vi "optionsAcq_spectrumSmoothing.vi"(0 "reference":refnum<class "OSA300.lvclass">, 2 "smoothing":T1, 4 "readWrite":enum16{"read", "write"}(ring), 5 "error in (no error)":errorcluster, 6 "width":u16, 7 "ignore range violation (false)":bool, 8 "nrOfPasses":u16) -> (10 "nrOfPasses out":u16, 12 "width out":u16, 14 "duplicate reference":refnum<class "OSA300.lvclass">, 15 "status":string, 16 "smoothing out":T1, 19 "error out":errorcluster)   [LabVIEW 2010, in "OSA300.lvclass"]
uses:
  OSA300.lvclass
  _misc/Thorlabs_FTS_misc.llb/interferogram_smoothing.ctl
  OSA.lvclass
  OSA300.lvclass/OSA300.ctl
  _OSAchannel_class/OSAchannel.lvclass
  _dll/LVLib/FTSLib.lvlib
  OSA20X_misc.lvlib
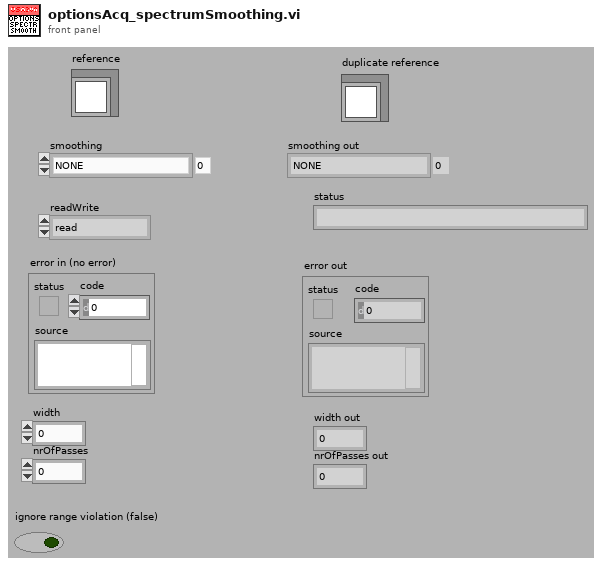
[diagram p1: front panel]
types:
  T1 = typedef "OSA20X_misc.lvlib/interferogram_smoothing.ctl" = enum16{"NONE", "BINOMIAL", "SAVITSKY_GOLAY", "FOURIER", "MOVING_AVERAGE", "GAUSSIAN"}
  T2 = typedef "OSA20X_misc.lvlib/channelType_spectrum.ctl" = enum16{"SINGLE CHANNEL", "STICHED"}
  T3 = typedef "OSA20X_misc.lvlib/amplifier_sort.ctl" = enum16{"amp_unknown", "amp_se_8", "amp_se_12_lg", "amp_se_12", "amp_se_16", "amp_diff_8", "amp_diff_12_lg", "amp_diff_12_ir", "amp_diff_16", "amp_other", "amp_other_2"}
  T4 = typedef "OSA20X_misc.lvlib/detector_sort.ctl" = enum16{"unknown", "Silicon", "Silicon PIN", "Silicon MPPC", "InGaAs", "InGaAs ext low", "InGaAs ext high", "InAs", "InAsSb", "InSb", "MCT", "other", "other2", "other3"}
  T5 = typedef "OSA20X_misc.lvlib/PDTemperatureMode.ctl" = enum16{"cool: better sensitivity/noise floor", "warm: extended wl range"}
  T6 = cluster{"waveMin (cm-1)":sgl, "waveMax (cm-1)":sgl, "gainOffset_auto":bool, "gain":i32, "gain levels nr":u16, "offset":i32, "offset max":u16, "damper available":bool, "damper active":bool, "amplifier sort":T3, "detector sort":T4, "channelIdx global":u16, "spectrIdx":u16, "waveMeter on":bool, "ref gainLevels rel.":refnum<data-value>, "intfgrm_smooth_width":u16, "intfgrm_smooth_nrOfPasses":u16, "intfgrm_smooth":T1, "adc #bits":u16, "temp Variable":bool, "spectr_smooth":T1, "spectr_smooth_width":u16, "spectr_smooth_nrOfPasses":u16, "PD sensitivity mode":T5}
  T7 = typedef "OSA.lvclass/ObjectAttributes.ctl" = cluster{"Stop":bool, "dataType":T8, "spectrometerIdx":u16, "buffer size interferogram":i32, "interferogram":cluster{"new":bool, "plot_x_ min":sgl, "plot_x_max":sgl, "plot_y_min":sgl, "plot_y_max":sgl, "Graph Intrfrgrm":T9, "timeStamp":u32, "signal (%)":dbl, "traces":cluster{"idx":u32, "broadBand":bool, "monoChromatic":bool, "peakToPeakSignal":dbl, "peakToPeakPos":dbl}[], "traces idx last":i32}, "spectrum":cluster{"new":bool, "plot_x_min":sgl, "plot_x_max":sgl, "plot_unit_x":T10, "plot_unit_y":T11, "plot_y_min":sgl, "plot_y_max":sgl, "Graph Spectrum":T9, "timeStamp":u32, "X_VAL_OPTIONS":enum16{"MIN_MAX", "ARRAY"}, "traces":cluster{"idx":u32}[], "traces idx last":i32}, "Thorlabs_OSA_64.lvclass:queue_action.ctlqueue ref":refnum<queue>, "action":T12, "plot zoom step":dbl, "buffer semaphore":T13, "acq stopped":bool, "dataType active":T8, "temperature (degr C)":sgl, "pressure (hPa)":sgl, "rel humidity (%)":sgl, "settings":cluster{"resolution":T14, "sensitivity":T15, "Average":bool, "average nr":u32, "apodisation":T16, "acq delay (ms)":u32, "airMesure":T17, "wmtr on":bool, "intfgrm_smooth_width":u16, "intfgrm_smooth_nrOfPasses":u16, "intfgrm_smooth":T1, "phaseCorrection":T18, "zeroFill":u8, "spectr_smooth":T1, "spectr_smooth_width":u16, "spectr_smooth_nrOfPasses":u16, "resolution (/cm)":sgl, "REF wavelength, (nm)":dbl, "gain_idx":u16, "gainAuto":bool, "gain_relative":dbl, "PD sensitivity mode":T5, "PD senseMode implemented":bool, "SensorTemperature implemented":bool, "SensorPressure implemented":bool, "SensorHumidity implemented":bool}, "peaks position":sgl[], "peaks width":sgl[], "peaks height":sgl[], "peaks max nr":u32, "peaks latest nr":i32, "peaks new":bool, "power":dbl, "power new":bool, "path":string, "wavelength (WNr)":dbl, "wavelength new":bool, "buffer size spectrum":i32, "status":string, "VI reference":refnum<vi>, "funcPointer":u64, "libraryPointer":u64, "singleAcquisition":bool, "coherenceLength (cm)":dbl, "coherenceLength new":bool, "spectrometer model":string, "spectrometer serial nr":string, "peaks thld left":sgl[], "peaks thld right":sgl[], "coherenceLength error (cm)":dbl, "ADC bits":u16, "peaks position centroid":sgl[], "peaks height centroid":sgl[], "OSA series":T19, "channel index spectrum":u16, "spectrometer rangeLow, (/cm)":dbl, "spectrometer rangeHigh, (/cm)":dbl, "channel index interferogram":u16}
  T8 = typedef "OSA.lvclass/acq_dataType.ctl" = enum16{"none", "interferogram", "spectrum"}
  T9 = typedef "OSA.lvclass/graph_intensity.ctl" = refnum<vi>
  T10 = typedef "OSA.lvclass/spectrum_x_unit.ctl" = enum16{"wavenr/cm", "THz", "eV", "nm_air", "nm_vac"}
  T11 = typedef "OSA.lvclass/y_unit.ctl" = enum16{"ADC counts", "dBm pwr absolute", "dBm pwr density", "mW pwr absolute", "mW pwr density"}
  T12 = typedef "OSA.lvclass/queue_action.ctl" = enum16{"none", "stop", "GUI_plotInterferogram", "GUI_plotSpectrum", "GUI_plotInterferogramRescale", "GUI_plotSpectrumRescale", "GUI_plotInterferogramReset", "GUI_plotSpectrumReset", "GUI_plotInterferogramAutoScaleY", "GUI_plotSpectrumAutoScaleY", "GUI_plotInterferogramZoomOut", "GUI_plotSpectrumZoomOut", "GUI_plotInterferogramPane", "GUI_plotSpectrumPane", "GUI_plotInterferogramZoomMouse", "GUI_plotSpectrumZoomMouse", "ENVIRONMENT temperature", "ENVIRONMENT pressure", "MODE_resolution set", "MODE_resolution get", "MODE_sensitivity set", "MODE_sensitivity get", "MODE_PDTemperature set", "MODE_PDTemperature get", "REBOOT/RESET firmware", "ACQASYNC_acquireSingleSpectrum", "ACQASYNC_continuous start", "ACQASYNC_continuous stop\n", "ACQASYNC_get last interferogram", "ACQASYNC_get last spectrum", "ACQASYNC_get last waveNr", "ACQOPT_interferogram smoothing set", "ACQOPT_interferogram smoothing get", "ACQOPT_spectrum smoothing set", "ACQOPT_spectrum smoothing get", "ACQOPT_apodisation type set", "ACQOPT_apodisation type get", "ACQOPT_phase correction type set", "ACQOPT_phase correction type get", "ACQOPT_acqIntervall_set", "ACQOPT_acqIntervall_get", "ACQOPT_average spectrum set", "ACQOPT_average spectrum get", "ACQOPT_rolling average set", "ACQOPT_rolling average get", "ACQOPT_zero fill factor set", "ACQOPT_zero fill factor get", "ACQOPT_cycle counting set", "ACQOPT_cycle counting get", "ACQOPT_air measure option set", "ACQOPT_air measure option get", "ACQOPT_gainLevel auto get", "ACQOPT_gainLevel auto set", "ACQOPT_gainLevel get", "ACQOPT_gainLevel set", "ACQOPT_getAll", "INSTRUMENT_PROPERTY_range_WaveNr_min", "INSTRUMENT_PROPERTY_range_WaveNr_max", "INSTRUMENT_PROPERTY_reference_wavelength_cm^-1", "INSTRUMENT_PROPERTY_samplesPerRefPeriod", "INSTRUMENT_PROPERTY_resolution_waveNrPercm", "INSTRUMENT_PROPERTY_availableGainLevels", "INSTRUMENT_PROPERTY_status", "CONVERT", "ANALYSE_POWER", "ANALYSE_PEAKS", "ANALYSE_WAVELENGTH", "ANALYSE_SPECTRUM", "ANALYSE_INTERFEROGRAM", "ANALYSE_COHERENCE_LENGTH", "MATH", "MATH_power", "MATH_peaks", "FILE", "miscellaneous"}
  T13 = typedef "Semaphore RefNum" = refnum<k1>
  T14 = typedef "OSA.lvclass/resolution.ctl" = enum16{"low", "high"}
  T15 = typedef "OSA.lvclass/sensitivityMode.ctl" = enum16{"low", "low medium", "high medium", "high"}
  T16 = typedef "OSA.lvclass/apodisation.ctl" = enum16{"NONE", "NORTON_BEER_WEAK", "NORTON_BEER_MEDIUM", "NORTON_BEER_STRONG", "TRIANGULAR", "COSINE", "HANN", "HAMMING", "BLACKMANHARRIS3", "BLACKMANHARRIS4", "GAUSSIAN"}
  T17 = typedef "OSA.lvclass/airMeasure.ctl" = enum16{"TEMPERATURE", "PRESSURE"}
  T18 = typedef "OSA.lvclass/phaseCorrection.ctl" = enum16{"NONE", "MERTZ", "FORMAN", "MERTZ_FILE", "FORMAN_FILE", "FUTURE COMP."}
  T19 = typedef "OSA.lvclass/OSA_series.ctl" = enum16{"OSA200", "OSA300", "UNKNOWN"}
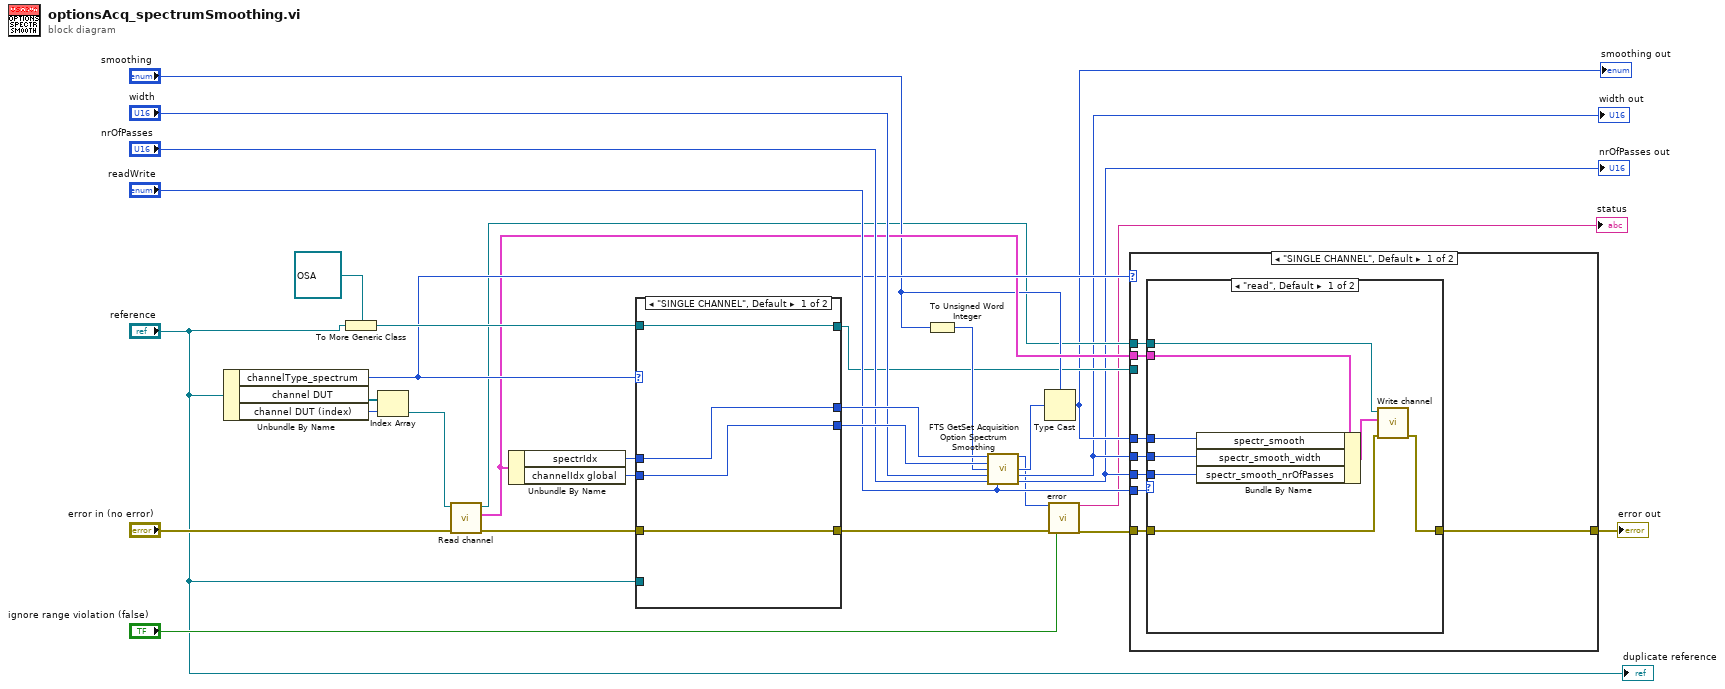
[diagram p0: block diagram]
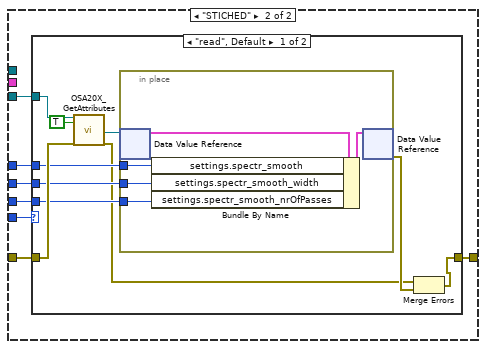
[diagram p3: hidden frame]
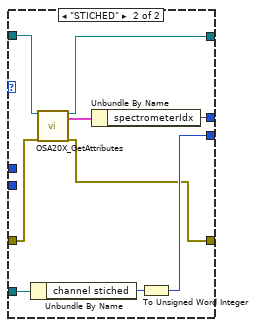
[diagram p5: hidden frame]
diagram:
  n1 = Unbundle By Name("reference") -> ("channelType_spectrum"=w21:T2, "channel DUT"=w23:refnum<class "OSAchannel.lvclass">[], "channel DUT (index)"=w22:i32)
  n2 = To More Generic Class(target class=refnum<class "OSA.lvclass"> refnum ("Thorlabs_OSA_64"), reference="reference") -> (generic class reference=w30:refnum<class "OSA.lvclass">)
  n3 = Index Array(array=w23, index=w22) -> (element=w20:refnum<class "OSAchannel.lvclass">)
  n4 = call "Read channel.vi"("error in (no error)"="error in (no error)", "OSAchannel in"=w20) -> ("error out"=w16:errorcluster, "channel"=w15:T6, "OSAchannel out"=w11:refnum<class "OSAchannel.lvclass">)  [unwired: 7 in]
  n5 = Unbundle By Name(w15) -> ("spectrIdx"=w19:u16, "channelIdx global"=w18:u16)
  n6 = case shown="\"SINGLE CHANNEL\", Default" w21 {
    tunnel: [w32 w39] -> w6
    tunnel: [w34 w43] -> w29
    tunnel: [w33 w42] -> w28
    tunnel: w16 -> [w32 w36]
    tunnel: w30 -> [w35 w41]
    tunnel: [w35 w40] -> w10
    tunnel: "reference" -> [_ w38]
    tunnel: w19 -> [w34 _]
    tunnel: w18 -> [w33 _]
    frame "SINGLE CHANNEL", Default {
    }
    frame "STICHED" {
      n7 = Unbundle By Name(w38) -> ("channel stiched"=w44:u32)
      n8 = call "OSA20X_GetAttributes.vi"("reference in"=w41, "error in (no error)"=w36) -> ("reference out"=w40:refnum<class "OSA.lvclass">, "Data"=w37:T7, "error out"=w39:errorcluster)  [unwired: 14 in, 1 out]
      n9 = Unbundle By Name(w37) -> ("spectrometerIdx"=w43:u16)
      n10 = To Unsigned Word Integer(number=w44) -> (unsigned 16bit integer=w42:u16)
    }
  }
  n11 = To Unsigned Word Integer(number="smoothing") -> (unsigned 16bit integer=w27:u16)
  n12 = call "FTS GetSet Acquisition Option Spectrum Smoothing.vi"("spectrIdx"=w29, "channel"=w28, "smoothingType"=w27, "width"="width", "nrOfPasses"="nrOfPasses", "readWrite"="readWrite") -> ("FTSLib status"=w4:i32, "smoothingType"=w13:u16, "width read"=w8:u16, "nrOfPAsses read"=w7:u16)  [unwired: 6 in]
  "nrOfPasses out" <- w7
  "width out" <- w8
  n13 = Type Cast(type="smoothing", x=w13) -> (*(type *) &x=w9:T1)
  "smoothing out" <- w9
  n14 = call "error.vi"("result code"=w4, "error in (no error)"=w6, "ignore range violation"="ignore range violation (false)") -> ("status"=→"status":string, "error out"=w5:errorcluster)  [unwired: 14 in, 1 out]
  n15 = case shown="\"SINGLE CHANNEL\", Default" w21 {
    tunnel: w5 -> [w52 w67]
    tunnel: "readWrite" -> [w51 w62]
    tunnel: w9 -> [w50 w66]
    tunnel: w8 -> [w49 w65]
    tunnel: w15 -> [w48 _]
    tunnel: w7 -> [w47 w64]
    tunnel: [w46 w63] -> w12
    tunnel: w11 -> [w45 _]
    tunnel: w10 -> [_ w68]
    frame "SINGLE CHANNEL", Default {
      n16 = case shown="\"read\", Default" w51 {
        tunnel: w52 -> [w60 w61]
        tunnel: w48 -> [w59 _]
        tunnel: w50 -> [w57 _]
        tunnel: w49 -> [w56 _]
        tunnel: w47 -> [w55 _]
        tunnel: [w54 w61] -> w46
        tunnel: w45 -> [w53 _]
        frame "read", Default {
          n17 = Bundle By Name(cluster=w59, "spectr_smooth"=w57, "spectr_smooth_width"=w56, "spectr_smooth_nrOfPasses"=w55) -> (w58:T6)
          n18 = call "Write channel.vi"("error in (no error)"=w60, "channel"=w58, "OSAchannel in"=w53) -> ("error out"=w54:errorcluster)  [unwired: 7 in, 1 out]
        }
        frame "write" {
        }
      }
    }
    frame "STICHED" {
      n19 = case shown="\"read\", Default" w62 {
        tunnel: w68 -> [w78 _]
        tunnel: w67 -> [w76 w84]
        tunnel: w66 -> [w74 _]
        tunnel: w65 -> [w73 _]
        tunnel: w64 -> [w72 _]
        tunnel: [w69 w84] -> w63
        frame "read", Default {
          n20 = call "OSA20X_GetAttributes.vi"("reference in"=w78, "OnlyGetDvrReference(False)"=TRUE, "error in (no error)"=w76) -> ("DataRef"=w75:refnum<data-value>, "error out"=w70:errorcluster)  [unwired: 13 in, 2 out]
          n21 = in-place {
            in-place-border: w74 -> [w81]
            in-place-border: w73 -> [w80]
            in-place-border: w72 -> [w79]
            n22 = in-place-dvr #1(w75) -> (w83:T7)  [unwired: 1 out]
            n23 = Bundle By Name(cluster=w83, "settings.spectr_smooth"=w81, "settings.spectr_smooth_width"=w80, "settings.spectr_smooth_nrOfPasses"=w79) -> (w82:T7)
            n24 = in-place-dvr #1(w82) -> (w71:errorcluster)  [unwired: 1 out]
          }
          n25 = Merge Errors(w70, w71) -> (w69:errorcluster)
        }
        frame "write" {
        }
      }
    }
  }
  "error out" <- w12
  "duplicate reference" <- "reference"
